vi "Power Spectrum (CDB).vi"(0 "X":cdb[](array[numeric])) -> (1 "Power Spectrum":dbl[](array[numeric]), 2 "error":i32)   [LabVIEW 2010, in "NI_AALPro.lvlib"]
doc: "Computes the <B>Power Spectrum</B>, Sxx, of the input sequence <B>X</B>. Wire data to the <B>X</B> input to determine the polymorphic instance to use or manually select the instance."
uses:
  NI_AALPro.lvlib
  lvanlys.dll
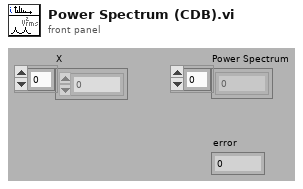
[diagram p1: front panel]
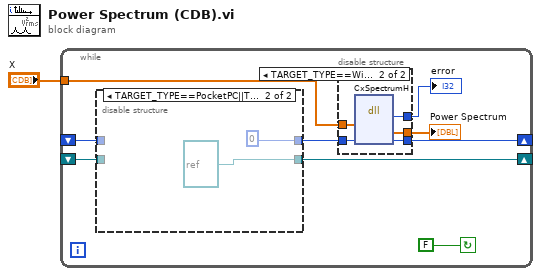
[diagram p0: block diagram]
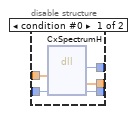
[diagram p2: hidden frame]
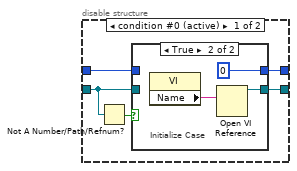
[diagram p3: hidden frame]
diagram:
  n1 = while {
    shift-left: _ -> [w7]
    shift-right: [w4] -> _
    tunnel: "X" -> [w10]
    shift-right: [w5] -> _
    shift-left: _ -> [w6]
    stop <- FALSE continue-if-true
    n2 = disable-structure shown="TARGET_TYPE==PocketPC||TARGET_TYPE==PalmOS||TARGET_TYPE==FPGA||TARGET_TYPE==Embedded" {
      disable-tunnel: w6 -> [w23 _]
      disable-tunnel: [w24 refnum<vi> refnum ("VI Refnum")] -> w5
      disable-tunnel: w7 -> [w22 _]
      disable-tunnel: [w21 0 ("t")] -> w3
      frame condition #0 (active) {
        n3 = Not A Number/Path/Refnum?(number/path/refnum=w23) -> (NaN/Path/Refnum?=w25:bool)
        n4 = case shown="True" w25 {
          tunnel: [w27 w29] -> w24
          tunnel: w23 -> [w27 _]
          tunnel: w22 -> [w26 _]
          tunnel: [w26 0 ("error")] -> w21
          frame False {
          }
          frame True {
            # "Initialize Case"
            n5 = property class="VI"() -> ("Name"=w28:string)  [unwired: 2 in, 2 out]
            n6 = Open VI Reference(vi path=w28) -> (vi reference=w29:refnum<vi>)  [unwired: 5 in, 1 out]
          }
        }
      }
      frame condition #1 {
      }
    }
    n7 = disable-structure shown="TARGET_TYPE==Windows||TARGET_TYPE==Mac||TARGET_TYPE==Unix" {
      disable-tunnel: w10 -> [w15 w20]
      disable-tunnel: [w14 w19] -> w9
      disable-tunnel: [w13 w18] -> w4
      disable-tunnel: w3 -> [w12 w17]
      disable-tunnel: [w11 w16] -> w2
      frame condition #0 {
        n8 = dll-call lib="C:/Program Files/National Instruments/LabVIEW 2010/resource/lvanlys.*" fn="CxSpectrumH"("X"=w15, "tbl"=w12) -> (w14:i32, "spectrumXH"=w11:dbl[], "tbl"=w13:i32)  [unwired: 5 in, 2 out]
      }
      frame condition #1 (active) {
        n9 = dll-call lib="C:/Program Files/National Instruments/LabVIEW 2010/resource/lvanlys.dll" fn="CxSpectrumH"("xH"=w20, "tbl"=w17) -> ("return type"=w19:i32, "spectrumXH"=w16:dbl[], "tbl"=w18:i64)  [unwired: 5 in, 2 out]
      }
    }
    "Power Spectrum" <- w2
    "error" <- w9
  }
